vi "Show Binary.vi"(0 "Input Image":T1(plugin-control), 5 "LUT1":cluster{u16, u16}(slide)={0, 4095} caption="Slide" scale=0.0..4095.0, 7 "Boundary":dbl, 11 "error in (no error)":errorcluster) -> (4 "Binary Image":T1(plugin-control), 6 "Reference Rectangles":i16[][](array[numeric]), 10 "Histogram Graph":T2 {"Incremental Value" format="%.2f"; "Starting Value" format="%.2f"}, 14 "Number of Particles":i32, 15 "error out":errorcluster)   [LabVIEW 2017]
uses:
  <vilib>/vision/Image Controls.llb/IMAQ Image.ctl
  <vilib>/vision/NI_Vision_Development_Module.lvlib
panel:
  out "got copy":bool=TRUE
  out "upper":u16
  out "lower":u16
  out "Mean Value":sgl format="%.2f"
  out "temp copy":T1
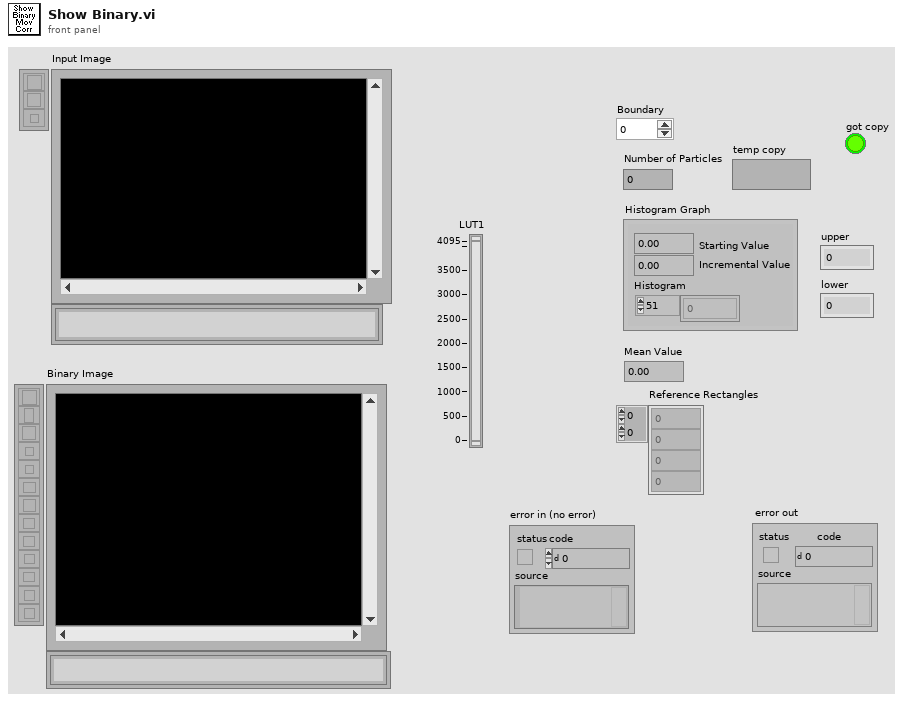
[diagram p1: front panel]
types:
  T1 = typedef "IMAQ Image.ctl" = refnum<image>
  T2 = cluster{"Starting Value":sgl, "Incremental Value":sgl, "Histogram":u32[]}
  T3 = cluster{"Left":i32, "Top":i32, "Right":i32, "Bottom":i32}
  T4 = typedef "Particle Parameters" = i32
  T5 = typedef "Image Type" = u32
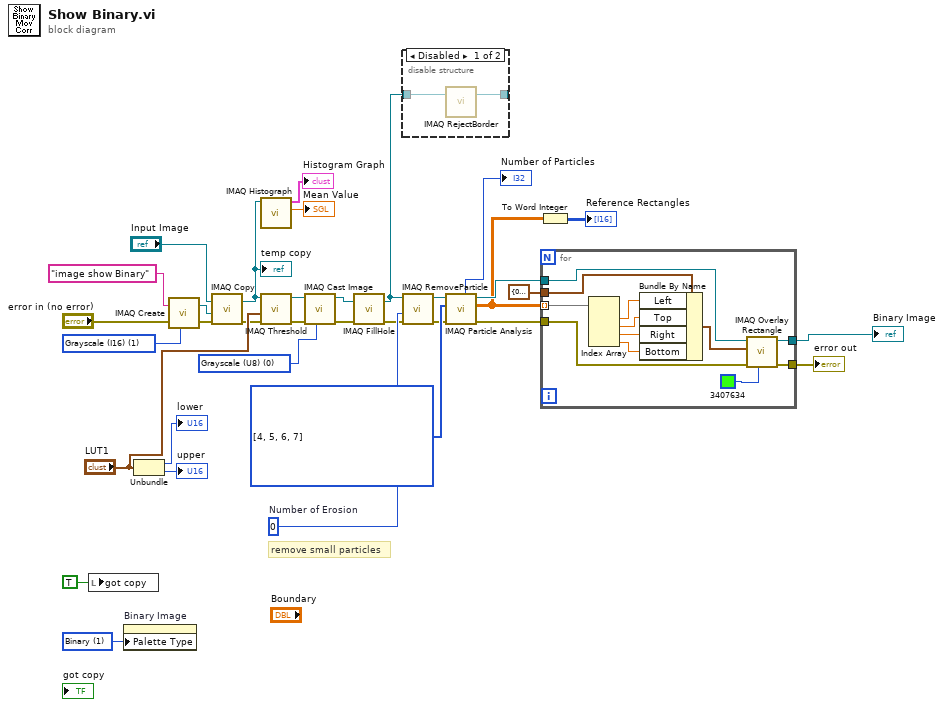
[diagram p0: block diagram]
diagram:
  w17 = u32 1 items=["Grayscale", "Binary", "Gradient", "Rainbow", "Temperature", "User Defined"] ("Palette:Palette Type")
  w23 = T4[] [4, 5, 6, 7] items=["Center of Mass X", "Center of Mass Y", "First Pixel X", "First Pixel Y", "Bounding Rect Left", "Bounding Rect Top", "Bounding Rect Right", "Bounding Rect Bottom", "Max Feret Diameter Start X", "Max Feret Diameter Start Y", "Max Feret Diameter End X", "Max Feret Diameter End Y", "Max Horiz. Segment Length Left", "Max Horiz. Segment Length Right", "Max Horiz. Segment Length Row", "-", "Bounding Rect Width", "Bounding Rect Height", "Bounding Rect Diagonal", "Perimeter", "Convex Hull Perimeter", "Holes' Perimeter", "Max Feret Diameter", "Equivalent Ellipse Major Axis", "Equivalent Ellipse Minor Axis", "Equivalent Ellipse Minor Axis (Feret)", "Equivalent Rect Long Side", "Equivalent Rect Short Side", "Equivalent Rect Diagonal", "Equivalent Rect Short Side (Feret)", "Average Horiz. Segment Length", "Average Vert. Segment Length", "Hydraulic Radius", "Waddel Disk Diameter", "-", "Area", "Holes' Area", "Particle & Holes' Area", "Convex Hull Area", "Image Area", "-", "Number of Holes", "Number of Horiz. Segments", "Number of Vert. Segments", "-", "Orientation", "Max Feret Diameter Orientation", "-", "% Area/Image Area", "% Area/(Particle & Holes' Area)", "Ratio of Equivalent Ellipse Axes", "Ratio of Equivalent Rect Sides", "-", "Elongation Factor", "Compactness Factor", "Heywood Circularity Factor", "Type Factor", "-", "Sum X", "Sum Y", "Sum XX", "Sum XY", "Sum YY", "Sum XXX", "Sum XXY", "Sum XYY", "Sum YYY", "-", "Moment of Inertia XX", "Moment of Inertia XY", "Moment of Inertia YY", "Moment of Inertia XXX", "Moment of Inertia XXY", "Moment of Inertia XYY", "Moment of Inertia YYY", "Norm. Moment of Inertia XX", "Norm. Moment of Inertia XY", "Norm. Moment of Inertia YY", "Norm. Moment of Inertia XXX", "Norm. Moment of Inertia XXY", "Norm. Moment of Inertia XYY", "Norm. Moment of Inertia YYY", "Hu Moment 1", "Hu Moment 2", "Hu Moment 3", "Hu Moment 4", "Hu Moment 5", "Hu Moment 6", "Hu Moment 7"] ("Pixel Measurements")
  w24 = 0  # Number of Erosion
  w25 = T5 0 items=["Grayscale (U8)", "Grayscale (I16)", "Grayscale (SGL)", "Complex (CSG)", "RGB (U32)", "HSL (U32)", "RGB (U64)", "Grayscale (U16)"] ("Image Type")
  w33 = T5 1 items=["Grayscale (U8)", "Grayscale (I16)", "Grayscale (SGL)", "Complex (CSG)", "RGB (U32)", "HSL (U32)", "RGB (U64)", "Grayscale (U16)"] ("Image Type")
  # "remove small particles"
  n1 = local write "got copy"(TRUE) -> ()
  n2 = property on="Binary Image" class="ImageControl"("Palette Type"=w17) -> ()  [unwired: 2 in, 2 out]
  n3 = Unbundle("LUT1") -> (→"lower":u16, →"upper":u16)
  n4 = call "IMAQ Create"("Image Name"="image show Binary", "Image Type"=w33, "error in (no error)"="error in (no error)") -> ("New Image"=w32:T1, "error out"=w4:errorcluster)  [unwired: 2 in]
  n5 = call "IMAQ Copy"("error in (no error)"=w4, "Image Dst"=w32, "Image Src"="Input Image") -> ("error out"=w5:errorcluster, "Image Dst Out"=w28:T1)  [unwired: 3 in]
  "temp copy" <- w28
  n6 = call "IMAQ Histograph"("Image"=w28) -> ("Mean Value"=→"Mean Value":sgl, "Histogram Graph"=→"Histogram Graph":T2)  [unwired: 7 in, 2 out]
  n7 = call "IMAQ Threshold"("error in (no error)"=w5, "Range"="LUT1", "Image Src"=w28) -> ("error out"=w6:errorcluster, "Image Dst Out"=w27:T1)  [unwired: 3 in, 4 out]
  n8 = call "IMAQ Cast Image"("Image Type"=w25, "error in (no error)"=w6, "Image Src"=w27) -> ("error out"=w7:errorcluster, "Image Dst Out"=w26:T1)  [unwired: 7 in]
  n9 = call "IMAQ FillHole"("error in (no error)"=w7, "Image Src"=w26) -> ("error out"=w8:errorcluster, "Image Dst Out"=w16:T1)  [unwired: 2 in, 2 out]
  n10 = disable-structure shown="Disabled" {
    disable-tunnel: w16 -> [w36 _]
    disable-tunnel: [w35 _] -> _
    frame Disabled {
      n11 = call "IMAQ RejectBorder"("Image Src"=w36) -> ("Image Dst Out"=w35:T1)  [unwired: 3 in, 3 out]
    }
    frame Enabled {
    }
  }
  n12 = call "IMAQ RemoveParticle"("error in (no error)"=w8, "Number of Erosion"=w24, "Image Src"=w16) -> ("error out"=w9:errorcluster, "Image Dst Out"=w15:T1)  [unwired: 4 in, 3 out]
  n13 = call "IMAQ Particle Analysis"("error in (no error)"=w9, "Pixel Measurements"=w23, "Image"=w15) -> ("error out"=w10:errorcluster, "Particle Measurements (Pixels)"=w2:dbl[][], "Image Out (duplicate)"=w22:T1, "Number of Particles"=→"Number of Particles":i32)  [unwired: 3 in, 2 out]
  n14 = To Word Integer(number=w2) -> (16bit integer=→"Reference Rectangles":i16[][])
  n15 = for {
    tunnel: [w39] -> w13
    tunnel: w22 -> [w47]
    tunnel: w2 -> [w45] mode=indexing
    tunnel: T3 {"Left"=0, "Top"=0, "Right"=0, "Bottom"=0} ("Rectangle") -> [w46]
    tunnel: [w38] -> w11
    tunnel: w10 -> [w37]
    n16 = Index Array(array=w45) -> (element #1=w43:dbl, element #2=w42:dbl, element #3=w41:dbl, element #4=w40:dbl)  [unwired: 4 in]
    n17 = Bundle By Name(cluster=w46, "Left"=w43, "Top"=w42, "Right"=w41, "Bottom"=w40) -> (w44:T3)
    n18 = call "IMAQ Overlay Rectangle"("Color"=u32 3407634 ("Text Color (black)"), "error in (no error)"=w37, "Rectangle"=w44, "Image"=w47) -> ("error out"=w38:errorcluster, "Image Out"=w39:T1)  [unwired: 6 in]
  }
  "Binary Image" <- w13
  "error out" <- w11
